vi "ReadConfig.vi"(8 "error in (no error)":errorcluster, 11 "GRMActor in":refnum<class "FlatField.lvclass">) -> (0 "error out":errorcluster, 3 "GRMActor out":refnum<class "FlatField.lvclass">)   [LabVIEW 2020]
uses:
  FlatField.lvclass
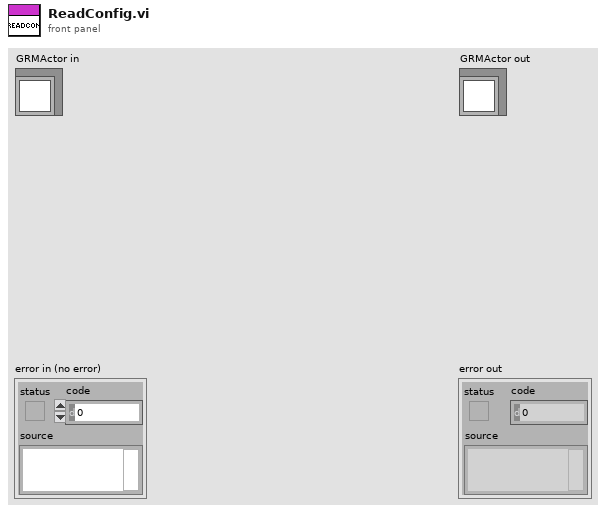
[diagram p1: front panel]
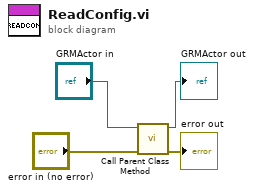
[diagram p0: block diagram]
diagram:
  n1 = call-parent "Call Parent Class Method"("error in (no error)"="error in (no error)", "GRMActor in"="GRMActor in") -> ("error out"=→"error out":errorcluster, "GRMActor out"=→"GRMActor out":refnum<class "FlatField.lvclass">)  [unwired: 8 in]
